vi "New2006.vi"   [LabVIEW 2013]
uses:
  <vilib>/Heliosphere Research LLC/Advanced Plotting Toolkit/api_core/NewPlotScales.ctl
  <vilib>/Heliosphere Research LLC/Advanced Plotting Toolkit/api_core/NewPlotType.ctl
  ErrorCodes.ctl
  <vilib>/Heliosphere Research LLC/Advanced Plotting Toolkit/Advanced Plotting Toolkit.lvlib
types:
  T1 = typedef "ErrorCodes.ctl" = u32
  T2 = typedef "Advanced Plotting Toolkit.lvlib/NewPlotType.ctl" = enum16{"Rectangular Axes", "Polar Axes"}
  T3 = typedef "Advanced Plotting Toolkit.lvlib/NewPlotScales.ctl" = enum16{"Default", "Linear", "Log", "Symlog"}
  T4 = typedef "Advanced Plotting Toolkit.lvlib/PlotID.ctl" = i32
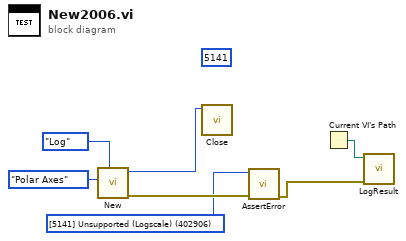
[diagram p0: block diagram]
diagram:
  w1 = T1 402906 items=["[5120] Invalid ID"=402902, "[5110] Failed to Init"=402900, "[5111] Unknown Error"=402901, "[5130] Save - Bad File Extension"=402403, "[5131] Save - General Error"=402904, "[5140] Unsupported (Polar)"=402905, "[5141] Unsupported (Logscale)"=402906, "[5142] Coordinates Not Regular"=402907] ("Expected Error")
  (unwired) 5141 ("Expected Error")
  n1 = call <vilib>:"New.vi"("X Axis Scale"=NewPlotScales."Log", "Plot Type"=NewPlotType."Polar Axes") -> ("error out"=w3:errorcluster, "Plot ID"=w4:T4)  [unwired: 8 in]
  n2 = call <vilib>:"Close.vi"("Plot ID"=w4) -> ()  [unwired: 10 in, 1 out]
  n3 = call "AssertError.vi"("error in (no error)"=w3, "Expected Error"=w1) -> ("error out"=w2:errorcluster)  [unwired: 9 in]
  n4 = Current VI's Path() -> (path=w7:path)
  n5 = call "LogResult.vi"("Test Result"=w2, "VI Path"=w7) -> ()  [unwired: 10 in]
